vi "meanT.vi"() -> ()   [LabVIEW 2019]
uses:
  <vilib>/Analysis/baseanly.llb/Mean (DBL).vi
  <vilib>/ptbypt/NI_PtbyPt.lvlib
  <vilib>/Analysis/NI_AALBase.lvlib
  <vilib>/gmath/NI_Gmath.lvlib
panel:
  out "mean value":dbl
  out "mean 2":dbl format="%0.2f"
  out "mean":dbl format="%0.2f"
  out "公分":dbl(slide) scale=0.0..200.0
  in  "stop":bool
  out "Waveform Chart":T1(graph)
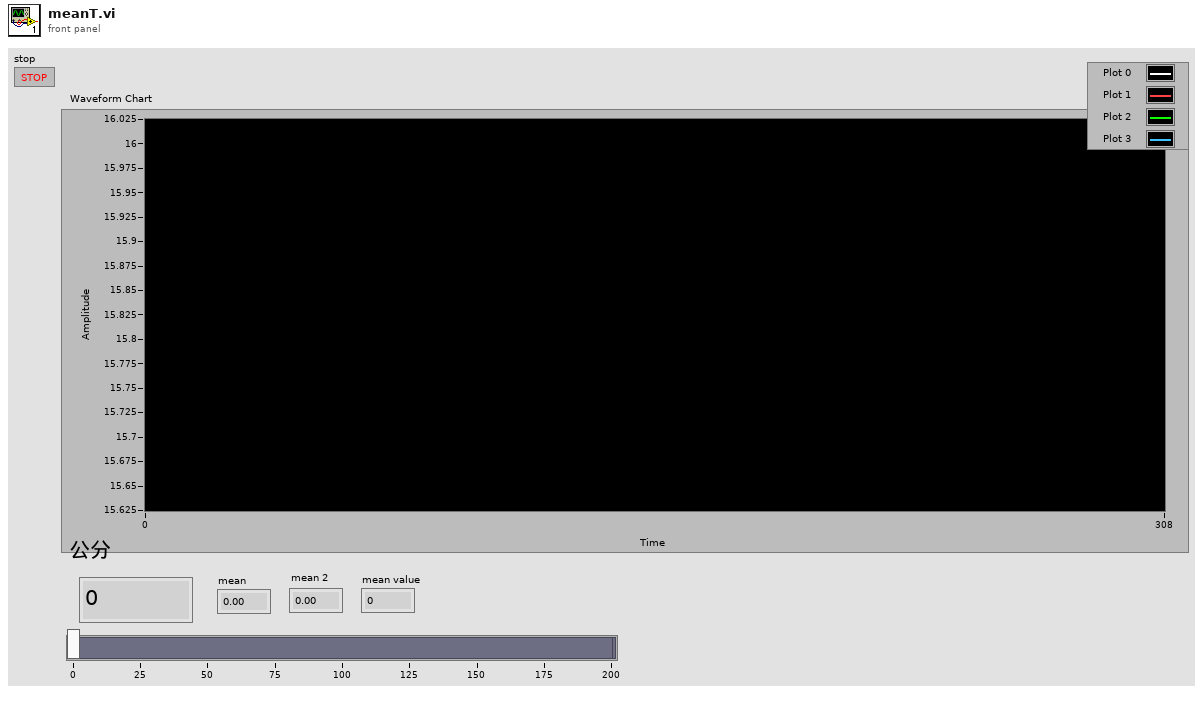
[diagram p1: front panel]
types:
  T1 = cluster{"公分":dbl, "mean":dbl, "mean":dbl, "mean value":dbl}
  T2 = enum16{"arithmetic", "geometric", "harmonic", "trimmed", "median"}
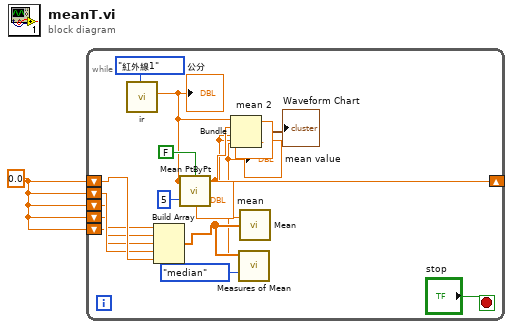
[diagram p0: block diagram]
diagram:
  w1 = 0.0 ("公分")
  n1 = while {
    shift-right: [w14] -> _
    shift-left: w1 -> [w12]
    shift-left: w1 -> [w11]
    shift-left: w1 -> [w10]
    shift-left: w1 -> [w9]
    shift-left: w1 -> [w8]
    stop <- "stop" stop-if-true
    n2 = call "ir.vi"("選擇紅外線"=enum16{"請選擇紅外線", "紅外線1", "紅外線2", "紅外線3", "紅外線4"}."紅外線1") -> ("公分"=w14:dbl)  [unwired: 9 in, 1 out]
    "公分" <- w14
    n3 = Build Array(w8, w9, w10, w11, w12) -> (w6:dbl[])
    n4 = call <vilib>:"Mean PtByPt.vi"("x"=w14, "sample length"=5, "initialize"=FALSE) -> ("mean"=w15:dbl)  [unwired: 1 in, 1 out]
    "mean" <- w15
    n5 = call <vilib>:"Measures of Mean.vi"("type"=T2."median", "x array"=w6) -> ("mean value"=w4:dbl)  [unwired: 8 in, 1 out]
    "mean value" <- w4
    n6 = call-poly <vilib>:"Mean.vi"("X"=w6) -> ("mean"=w7:dbl)  [unwired: 1 out]
    "mean 2" <- w7
    n7 = Bundle("公分"=w14, "mean"=w15, "mean"=w7, "mean value"=w4) -> (→"Waveform Chart":T1)  [unwired: 1 in]
  }
